vi "Shut Down Device.vi"(8 "error in (no error)":errorcluster, 11 "Virtual Camera in":refnum<class "Virtual Camera.lvclass">) -> (0 "error out":errorcluster, 3 "Virtual Camera out":refnum<class "Virtual Camera.lvclass">)   [LabVIEW 2015, in "Virtual Camera.lvlib" / "Virtual Camera.lvclass"]
uses:
  Virtual Camera.lvclass
  Camera/Camera.lvclass
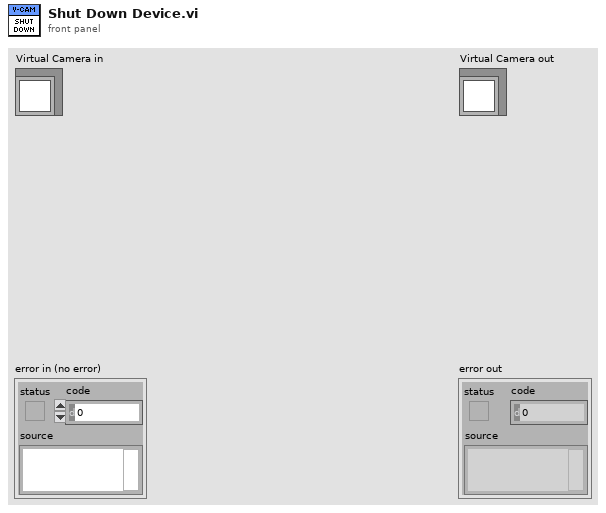
[diagram p1: front panel]
types:
  T1 = typedef "Camera Type.ctl" = enum16{"Orca-Flash 4.0 V2"}
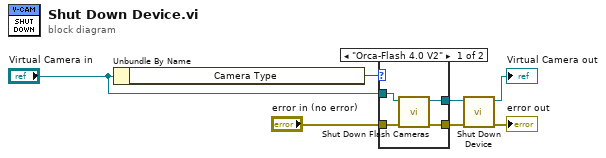
[diagram p0: block diagram]
diagram:
  n1 = Unbundle By Name("Virtual Camera in") -> ("Camera Type"=w5:T1)
  n2 = case shown="\"Orca-Flash 4.0 V2\"" w5 {
    tunnel: "Virtual Camera in" -> [w9 w13]
    tunnel: "error in (no error)" -> [w11 w12]
    tunnel: [w10 w12] -> w2
    tunnel: [w8 w13] -> w1
    frame "Orca-Flash 4.0 V2" {
      n3 = call-dynamic "Shut Down Flash Cameras.vi"("error in (no error)"=w11, "Virtual Camera in"=w9) -> ("error out"=w10:errorcluster, "Virtual Camera out"=w8:refnum<class "Virtual Camera.lvclass">)  [unwired: 8 in]
    }
    frame Default {
    }
  }
  n4 = call-parent "Shut Down Device.vi"("error in (no error)"=w2, "Device in"=w1) -> ("error out"=→"error out":errorcluster, "Device out"=→"Virtual Camera out":refnum<class "Virtual Camera.lvclass">)  [unwired: 8 in]
